vi "Parse Text.vi"(8 "Error In":errorcluster) -> (0 "Error Out":errorcluster)   [LabVIEW 2017, in "Tests.lvlib" / "Parser.lvlib"]
uses:
  Parser.lvlib
  src/Mustache/Public/Tokens/Public/Text/Text.lvclass
  src/Mustache/Public/Readers/Public/String/String.lvclass
  D:/Users/cfield/Code/Field R&D Services/Mustache/feature-lv-original-parser/src/Mustache/Public/Readers/Public/Abstract/Abstract.lvclass
  <vilib>/addons/_JKI Toolkits/Caraya/classes/Test/Test.lvclass
  src/Mustache/Public/Parser/Parser.lvclass
  <vilib>/addons/_JKI Toolkits/Caraya/classes/Assert/Assert.lvclass
  src/Mustache/Public/Tokens/Public/Abstract/Abstract.lvclass
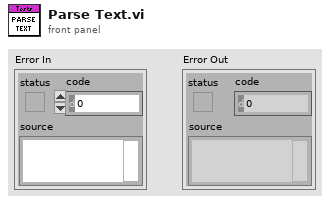
[diagram p1: front panel]
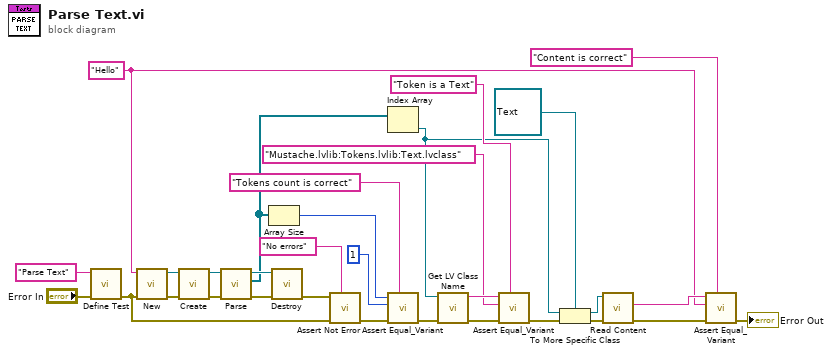
[diagram p0: block diagram]
diagram:
  w3 = "Hello" ("String")
  n1 = call <vilib>:"Define Test.vi"("error in (no error)"="Error In", "Label (VI Title)"="Parse Text") -> ("error out"=w22:errorcluster)  [unwired: 9 in]
  n2 = call "New.vi"("Error In"=w22, "String"=w3) -> ("Error Out"=w28:errorcluster, "String"=w29:refnum<class "String.lvclass">)  [unwired: 8 in]
  n3 = call "Create.vi"("Error In"=w28, "Reader"=w29) -> ("Error Out"=w27:errorcluster, "Parser"=w26:refnum<class "Parser.lvclass">)  [unwired: 8 in]
  n4 = call "Parse.vi"("Error In"=w27, "Parser In"=w26) -> ("Error Out"=w24:errorcluster, "Tokens"=w16:refnum<class "Abstract.lvclass">[], "Parser Out"=w25:refnum<class "Parser.lvclass">)  [unwired: 7 in]
  n5 = Array Size(array=w16) -> (size(s)=w18:i32)
  n6 = call "Destroy.vi"("Error In"=w24, "Parser"=w25) -> ("Error Out"=w23:errorcluster)  [unwired: 9 in]
  n7 = call <vilib>:"Assert Not Error.vi"("Label"="No errors", "error in (no error)"=w22, "Not Error?"=w23) -> ("error out"=w20:errorcluster)  [unwired: 8 in]
  n8 = Index Array(array=w16) -> (element=w10:refnum<class "Abstract.lvclass">)  [unwired: 1 in]
  n9 = call <vilib>:"Assert Equal_Variant.vi"("Label"="Tokens count is correct", "error in (no error)"=w20, "Y"=1 ("size(s)"), "X"=w18) -> ("error out"=w14:errorcluster)  [unwired: 7 in]
  n10 = call <vilib>:"Get LV Class Name.vi"("error in (no error)"=w14, "object"=w10) -> ("error out"=w13:errorcluster, "class name"=w12:string)  [unwired: 8 in]
  n11 = call <vilib>:"Assert Equal_Variant.vi"("Label"="Token is a Text", "error in (no error)"=w13, "Y"="Mustache.lvlib:Tokens.lvlib:Text.lvclass", "X"=w12) -> ("error out"=w9:errorcluster)  [unwired: 7 in]
  n12 = To More Specific Class(target class=refnum<class "Text.lvclass"> refnum ("Mustache.lvlib:Tokens.lvlib:Text.lvclass"), reference=w10, error in=w9) -> (specific class reference=w6:refnum<class "Text.lvclass">, error out=w7:errorcluster)
  n13 = call "Read Content.vi"("Error In"=w7, "Text In"=w6) -> ("Error Out"=w5:errorcluster, "Content"=w4:string)  [unwired: 7 in, 1 out]
  n14 = call <vilib>:"Assert Equal_Variant.vi"("Label"="Content is correct", "error in (no error)"=w5, "Y"=w3, "X"=w4) -> ("error out"=→"Error Out":errorcluster)  [unwired: 7 in]
